vi "SMTP Email [HELO].vi"(4 "error in (no error)":errorcluster, 7 "smtp session":T1) -> (0 "error out":errorcluster, 1 "reply":string, 2 "reply code":i32, 3 "smtp session out":T1)   [LabVIEW 2011, in "NewNI_SMTPEmail.lvlib"]
doc: "Sends a HELO command to the SMTP server through TCP connection described by \"SMTP Session\" and receives reply from the server."
uses:
  NewNI_SMTPEmail.lvlib
  SMTP Email Session.ctl
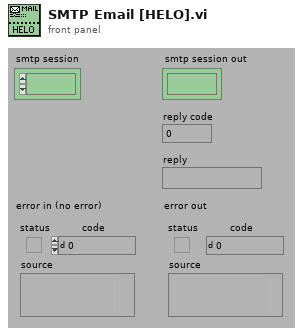
[diagram p1: front panel]
types:
  T1 = typedef "NewNI_SMTPEmail.lvlib/SMTP Email Session.ctl" = refnum<k1>
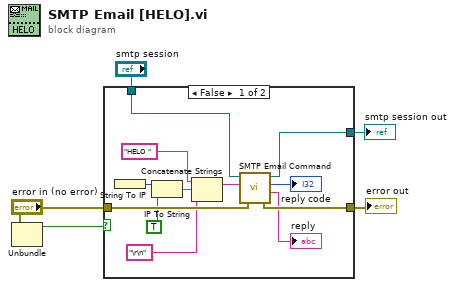
[diagram p0: block diagram]
diagram:
  n1 = Unbundle("error in (no error)") -> ("status"=w1:bool)  [unwired: 2 out]
  n2 = case shown="False" w1 {
    tunnel: "smtp session" -> [w15 w19]
    tunnel: [w14 w19] -> w4
    tunnel: [w12 w18] -> w3
    tunnel: "error in (no error)" -> [w11 w18]
    frame False {
      n3 = String To IP() -> (0:w13:u32)  [unwired: 1 out]
      n4 = IP To String(1:TRUE ("dot notation? (F)"), 2:w13) -> (0:w16:string)
      n5 = Concatenate Strings("HELO " ("HELO"), w16, "\r\n" ("HELO")) -> (w8:string)
      n6 = call "SMTP Email Command.vi"("error in (no error)"=w11, "command"=w8, "smtp session"=w15) -> ("error out"=w12:errorcluster, "reply"=→"reply":string, "reply code"=→"reply code":i32, "smtp session out"=w14:T1)  [unwired: 1 out]
    }
    frame True {
    }
  }
  "error out" <- w3
  "smtp session out" <- w4
